vi "Run greeter_server.vi"() -> ()   [LabVIEW 2019, in "helloworld_server.lvlib"]
uses:
  helloworld_server.lvlib
  RPC Service/Greeter/Greeter.lvclass
  C:/Program Files (x86)/National Instruments/LabVIEW 2019/vi.lib/gRPC/LabVIEW gRPC Servicer/ServiceBase/ServiceBase.lvclass
  <vilib>/gRPC/LabVIEW gRPC Servicer/Servicer/Servicer.lvclass/Servicer.ctl
  <vilib>/gRPC/LabVIEW gRPC Servicer/Servicer/Servicer.lvclass
panel:
  out "Listening Port":i32
  in  "Stop":bool
  in  "Server Address":string="localhost:50051"
  in  "Server Certificate File (.crt)":path
  in  "Server Key File (.key)":path
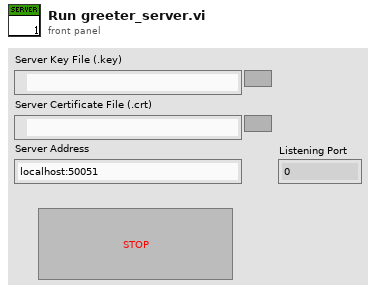
[diagram p1: front panel]
types:
  T1 = typedef "grpc-lvsupport-release.lvlib/grpcId.ctl" = u64
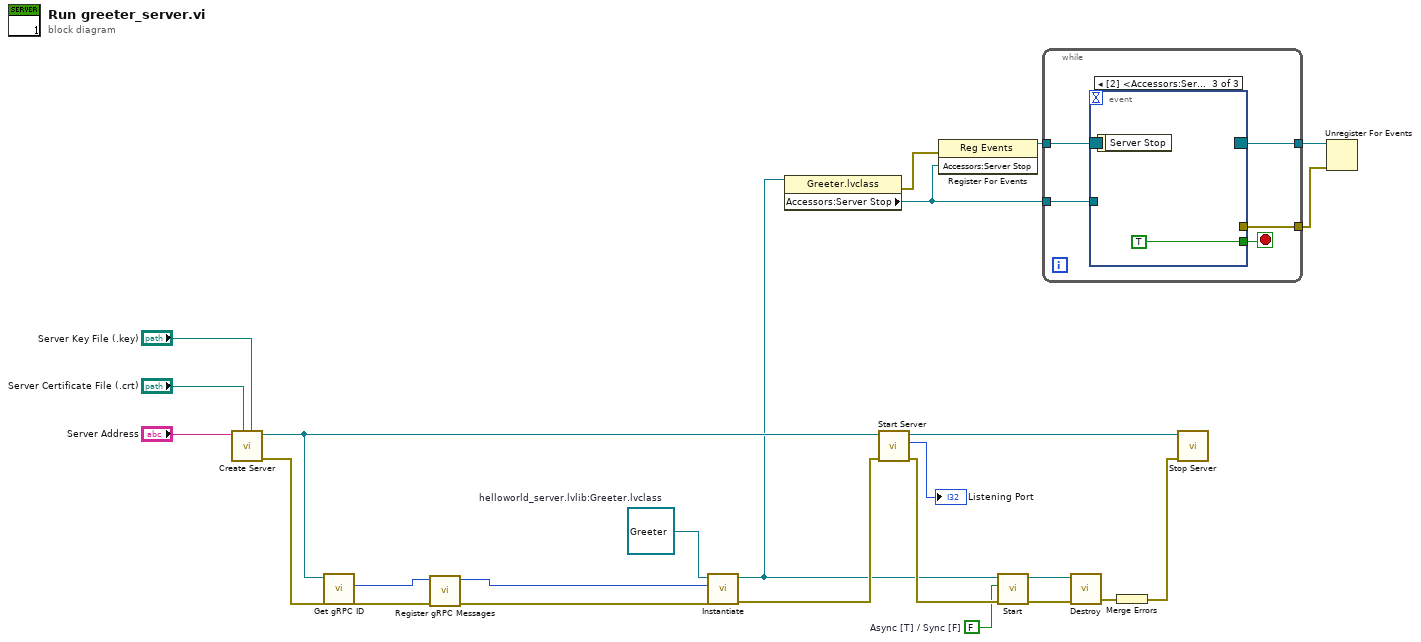
[diagram p0: block diagram]
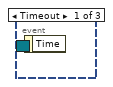
[diagram p2: hidden frame]
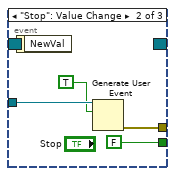
[diagram p3: hidden frame]
diagram:
  w4 = FALSE  # Async [T] / Sync [F]
  w1 = refnum<class "Greeter.lvclass"> refnum  # helloworld_server.lvlib:Greeter.lvclass
  n1 = call <vilib>:"Create Server.vi"("Server Key File (.key)"="Server Key File (.key)", "Server Certificate File (.crt)"="Server Certificate File (.crt)", "Server Address"="Server Address") -> ("error out"=w10:errorcluster, "gRPC Server out"=w17:refnum<class "Servicer.lvclass">)  [unwired: 7 in]
  n2 = call <vilib>:"Get gRPC ID.vi"("OOP Server in"=w17) -> ("gRPC ID"=w11:T1)  [unwired: 9 in, 1 out]
  n3 = call "Register gRPC Messages.vi"("error in (no error)"=w10, "gRPC ID"=w11) -> ("error out"=w9:errorcluster, "gRPC ID Out"=w8:T1)  [unwired: 8 in]
  n4 = call-dynamic "Instantiate.vi"("error in"=w9, "gRPCid"=w8, "iService"=w1) -> ("error out"=w15:errorcluster, "iService"=w3:refnum<class "Greeter.lvclass">)  [unwired: 7 in]
  n5 = property class="Greeter.lvclass"(reference=w3) -> (error out=w16:errorcluster, "Accessors:Server Stop"=w2:refnum<user-event>)  [unwired: 1 in, 1 out]
  n6 = call <vilib>:"Start Server.vi"("error in"=w15, "gRPC Server in"=w17) -> ("error out"=w7:errorcluster, "Listening Port"=→"Listening Port":i32, "gRPC Server out"=w24:refnum<class "Servicer.lvclass">)  [unwired: 7 in]
  n7 = register-events(error in=w16, w2) -> (reference out=w20:refnum<event-registration>)  [unwired: 1 in, 1 out]
  n8 = call-dynamic "Start.vi"("error in"=w7, "ASync [T]"=w4, "iService in"=w3) -> ("error out"=w6:errorcluster, "iService out"=w5:refnum<class "Greeter.lvclass">)  [unwired: 7 in]
  n9 = while {
    tunnel: w20 -> [w29]
    tunnel: [w27] -> w19
    tunnel: [w25] -> w12
    tunnel: w2 -> [w26]
    stop <- w28 stop-if-true
    n10 = event shown="[2] <Accessors:Server Stop>: User Event" {
      selector: w29 -> [_ _ _]
      dyn-events: [_ _ _] -> w27
      timeout: _ -> [_ _ _]
      tunnel: [_ FALSE TRUE] -> w28
      tunnel: w26 -> [_ w32 _]
      tunnel: [_ w30 _] -> w25
      event Timeout {
        n11 = event-data() -> ()  [unwired: 1 in, 1 out]
      }
      event "Stop": Value Change {
        n12 = event-data() -> ()  [unwired: 1 in, 1 out]
        n13 = Generate User Event(user event=w32, event data cluster=TRUE ("event data")) -> (error out=w30:errorcluster)  [unwired: 2 in, 1 out]
      }
      event User Event {
        n14 = event-data() -> ()  [unwired: 1 in, 1 out]
      }
    }
  }
  n15 = call-dynamic "Destroy.vi"("error in (no error)"=w6, "SignalGeneratorService in"=w5) -> ("error out"=w14:errorcluster)  [unwired: 8 in, 1 out]
  n16 = Merge Errors(w14) -> (w13:errorcluster)
  n17 = call <vilib>:"Stop Server.vi"("error in"=w13, "gRPC Server in"=w24) -> ()  [unwired: 9 in, 1 out]
  n18 = Unregister For Events(event registration refnum=w19, error in=w12) -> ()  [unwired: 1 out]
